vi "Close VISA.vi"() -> ()   [LabVIEW 2019]
panel:
  in  "dup VISA session":refnum<visa-resource-name>
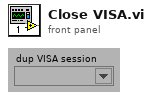
[diagram p1: front panel]
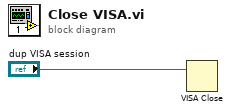
[diagram p0: block diagram]
diagram:
  n1 = VISA Close(VISA resource name="dup VISA session") -> ()  [unwired: 1 in, 1 out]
